vi "Write Actor Events.vi"(10 "Base Actor Events":T1, 11 "Template in":refnum<class "Template.lvclass">) -> (3 "Template out":refnum<class "Template.lvclass">)   [LabVIEW 2020, in "Template.lvlib" / "Template.lvclass"]
doc: "Sets the actor events cluster"
uses:
  Template.lvclass
  typedefs/base actor events.ctl
  typedefs/actor configuration.ctl
  typedefs/shared actor configuration.ctl
  typedefs/resource config/device configuration cluster.ctl
  typedefs/resource config/single resource cluster.ctl
  Template.lvclass/Template.ctl
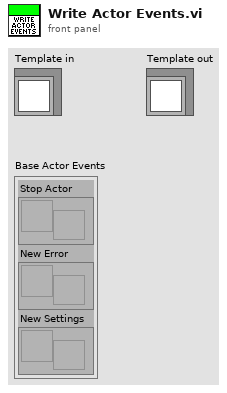
[diagram p1: front panel]
types:
  T1 = typedef "Template.lvlib/Template.lvclass/base actor events.ctl" = cluster{"Stop Actor":refnum<user-event>, "New Error":refnum<user-event>, "New Settings":refnum<user-event>}
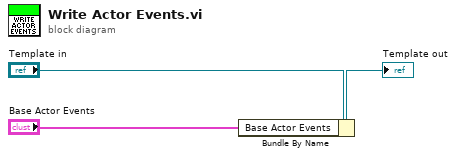
[diagram p0: block diagram]
diagram:
  n1 = Bundle By Name(cluster="Template in", "Base Actor Events"="Base Actor Events") -> (→"Template out":refnum<class "Template.lvclass">)
